vi "Finish.vi"   [LabVIEW 2015]
doc: "This VI is called just before exiting. It is expected to close I/O refnum, save collected data, etc."
uses:
  <vilib>/Rock Robotics/WPI/Utilities/WPI_GetSetVariantRefNum.vi
types:
  T1 = typedef "WPI_JoystickDevRef.ctl" = cluster{"Device":T2}
  T2 = typedef "WPI_JoystickDeviceEnum.ctl" = enum16{"USB 0", "USB 1", "USB 2", "USB 3", "USB 4", "USB 5"}
  T3 = typedef "WPI_CompressorDevRef.ctl" = cluster{"DevStatus":errorcluster, "Pneumatics Control Module":u8}
  T4 = typedef "WPI_EncoderDevRef.ctl" = cluster{"DevStatus":errorcluster, "EncoderIndex":T5, "CounterIndex":T6, "DistancePerCount":dbl, "Decoding Type":T7}
  T5 = typedef "FPGA_EncoderIdx.ctl" = enum8{"Enc 0", "Enc 1", "Enc 2", "Enc 3", "Enc 4", "Enc 5", "Enc 6", "Enc 7", "Invalid"}
  T6 = typedef "FPGA_CounterCtrSystemIndex.ctl" = enum8{"Ctr 0", "Ctr 1", "Ctr 2", "Ctr 3", "Ctr 4", "Ctr 5", "Ctr 6", "Ctr 7", "Invalid"}
  T7 = typedef "WPI_EncoderType.ctl" = enum16{"1x", "2x", "4x"}
  T8 = typedef "WPI_SolenoidDevRef.ctl" = cluster{"DevStatus":errorcluster, "Pneumatics Control Module":u8, "Forward Solenoid Channel":T9, "Reverse Solenoid Channel":T9}
  T9 = typedef "WPI_SolenoidChannel.ctl" = enum8{"Solenoid 0", "Solenoid 1", "Solenoid 2", "Solenoid 3", "Solenoid 4", "Solenoid 5", "Solenoid 6", "Solenoid 7", "Invalid"}
  T10 = typedef "WPI_ServoDeviceRef.ctl" = cluster{"DeviceStatus":errorcluster, "PWM Channel":T11, "DeadBand":T12}
  T11 = typedef "FPGA_DIOPWMChannel.ctl" = enum8{"PWM 0", "PWM 1", "PWM 2", "PWM 3", "PWM 4", "PWM 5", "PWM 6", "PWM 7", "PWM 8", "PWM 9", "PWM MXP 0", "PWM MXP 1", "PWM MXP 2", "PWM MXP 3", "PWM MXP 4", "PWM MXP 5", "PWM MXP 6", "PWM MXP 7", "PWM MXP 8", "PWM MXP 9", "Invalid"}
  T12 = typedef "WPI_PWMDeadband.ctl" = cluster{"Name":string, "maxPositivePwm":i32, "minPositivePwm":i32, "centerPwm":i32, "maxNegativePwm":i32, "minNegativePwm":i32, "angularRange":u16}
  T13 = typedef "WPI_SwitchDevRef.ctl" = cluster{"DevStatus":errorcluster, "DIO Channel":T14, "CntIndex":T6, "Normally Closed":bool}
  T14 = typedef "FPGA_DIOChannel.ctl" = enum8{"DIO 0", "DIO 1", "DIO 2", "DIO 3", "DIO 4", "DIO 5", "DIO 6", "DIO 7", "DIO 8", "DIO 9", "DIO MXP 0", "DIO MXP 1", "DIO MXP 2", "DIO MXP 3", "DIO MXP 4", "DIO MXP 5", "DIO MXP 6", "DIO MXP 7", "DIO MXP 8", "DIO MXP 9", "DIO MXP 10", "DIO MXP 11", "DIO MXP 12", "DIO MXP 13", "DIO MXP 14", "DIO MXP 15", "Invalid"}
  T15 = typedef "WPI_RobotDriveDevRef.ctl" = cluster{"DevStatus":errorcluster, "Motors[]":T16[], "Square Inputs":bool, "Max Output":dbl}
  T16 = typedef "WPI_MotorControlDeviceRef.ctl" = cluster{"DeviceStatus":errorcluster, "Type":T17, "PWM":cluster{"PWM Channel":T11, "DeadBand":T12}, "CAN":cluster{"Device Number":u8, "Control Mode":T18, "Semaphore":T19, "Max Vout":dbl, "TalonSRX Control Mode":T20}, "Invert":bool}
  T17 = typedef "WPI_MotorControlType.ctl" = enum16{"PWM", "CAN", "CANTalonSRX"}
  T18 = typedef "WPI_CANJaguar_ControlMode.ctl" = enum8{"Percent VBus", "Current", "Speed", "Position", "Voltage"}
  T19 = typedef "Semaphore RefNum" = refnum<k1>
  T20 = typedef "WPI_CANTalonSRX_APIControlMode.ctl" = enum8{"Percent VBus", "Speed", "Position", "Slave", "Unchanged / Invalid", "Voltage Compensation", "Current", "Motion Profile"}
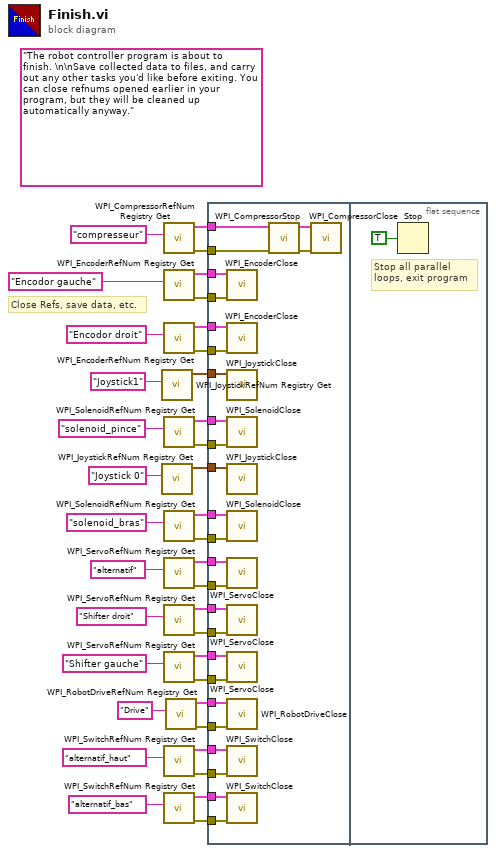
[diagram p0: block diagram]
diagram:
  (unwired) "The robot controller program is about to finish. \n\nSave collected data to files, and carry out any other tasks you'd like before exiting. You can close refnums opened earlier in your program, but they will be cleaned up automatically anyway."
  # "Close Refs, save data, etc."
  n1 = call <vilib>:"WPI_JoystickRefNum Registry Get.vi"("refnum name"="Joystick1") -> ("JoystickDevRef"=w22:T1)  [unwired: 1 in, 9 out]
  n2 = call <vilib>:"WPI_JoystickRefNum Registry Get.vi"("refnum name"="Joystick 0") -> ("JoystickDevRef"=w34:T1)  [unwired: 1 in, 9 out]
  n3 = call <vilib>:"WPI_CompressorRefNum Registry Get.vi"("refnum name"="compresseur") -> ("error out"=w16:errorcluster, "CompressorDevRef"=w17:T3)  [unwired: 9 in]
  n4 = call <vilib>:"WPI_EncoderRefNum Registry Get.vi"("refnum name"="Encodor gauche") -> ("error out"=w11:errorcluster, "EncoderDevRef"=w12:T4)  [unwired: 9 in]
  n5 = call <vilib>:"WPI_EncoderRefNum Registry Get.vi"("refnum name"="Encodor droit") -> ("error out"=w10:errorcluster, "EncoderDevRef"=w9:T4)  [unwired: 9 in]
  n6 = call <vilib>:"WPI_SolenoidRefNum Registry Get.vi"("refnum name"="solenoid_pince") -> ("error out"=w8:errorcluster, "SolenoidDevRef"=w18:T8)  [unwired: 9 in]
  n7 = call <vilib>:"WPI_SolenoidRefNum Registry Get.vi"("refnum name"="solenoid_bras") -> ("error out"=w7:errorcluster, "SolenoidDevRef"=w21:T8)  [unwired: 9 in]
  n8 = call <vilib>:"WPI_ServoRefNum Registry Get.vi"("refnum name"="alternatif") -> ("error out"=w1:errorcluster, "ServoDeviceRef"=w28:T10)  [unwired: 9 in]
  n9 = call <vilib>:"WPI_ServoRefNum Registry Get.vi"("refnum name"="Shifter droit") -> ("error out"=w6:errorcluster, "ServoDeviceRef"=w33:T10)  [unwired: 9 in]
  n10 = call <vilib>:"WPI_ServoRefNum Registry Get.vi"("refnum name"="Shifter gauche") -> ("error out"=w5:errorcluster, "ServoDeviceRef"=w32:T10)  [unwired: 9 in]
  n11 = call <vilib>:"WPI_SwitchRefNum Registry Get.vi"("refnum name"="alternatif_haut") -> ("error out"=w3:errorcluster, "SwitchDevRef"=w25:T13)  [unwired: 9 in]
  n12 = call <vilib>:"WPI_SwitchRefNum Registry Get.vi"("refnum name"="alternatif_bas") -> ("error out"=w4:errorcluster, "SwitchDevRef"=w24:T13)  [unwired: 9 in]
  n13 = call <vilib>:"WPI_RobotDriveRefNum Registry Get.vi"("refnum name"="Drive") -> ("error out"=w2:errorcluster, "RobotDriveDevRef"=w35:T15)  [unwired: 1 in, 8 out]
  n14 = flat-sequence {
    tunnel: w35 -> [w63]
    tunnel: w34 -> [w62]
    tunnel: w33 -> [w61]
    tunnel: w32 -> [w60]
    tunnel: w28 -> [w59]
    tunnel: w25 -> [w58]
    tunnel: w24 -> [w57]
    tunnel: w22 -> [w56]
    tunnel: w21 -> [w55]
    tunnel: w18 -> [w54]
    tunnel: w17 -> [w51]
    tunnel: w16 -> [w50]
    tunnel: w12 -> [w49]
    tunnel: w11 -> [w48]
    tunnel: w10 -> [w47]
    tunnel: w9 -> [w46]
    tunnel: w8 -> [w45]
    tunnel: w7 -> [w44]
    tunnel: w6 -> [w43]
    tunnel: w5 -> [w42]
    tunnel: w4 -> [w41]
    tunnel: w3 -> [w40]
    tunnel: w2 -> [w39]
    tunnel: w1 -> [w38]
    frame #0 {
      n15 = call <vilib>:"WPI_EncoderClose.vi"("error in (no error)"=w48, "EncoderDevRef"=w49) -> ()  [unwired: 9 in, 1 out]
      n16 = call <vilib>:"WPI_EncoderClose.vi"("error in (no error)"=w47, "EncoderDevRef"=w46) -> ()  [unwired: 9 in, 1 out]
      n17 = call <vilib>:"WPI_JoystickClose.vi"("JoystickDevRef"=w56) -> ()  [unwired: 11 out]
      n18 = call <vilib>:"WPI_SolenoidClose.vi"("error in (no error)"=w45, "SolenoidDevRef"=w54) -> ()  [unwired: 9 in, 1 out]
      n19 = call <vilib>:"WPI_JoystickClose.vi"("JoystickDevRef"=w62) -> ()  [unwired: 11 out]
      n20 = call <vilib>:"WPI_SolenoidClose.vi"("error in (no error)"=w44, "SolenoidDevRef"=w55) -> ()  [unwired: 9 in, 1 out]
      n21 = call <vilib>:"WPI_ServoClose.vi"("error in (no error)"=w38, "ServoDeviceRef"=w59) -> ()  [unwired: 9 in, 1 out]
      n22 = call <vilib>:"WPI_ServoClose.vi"("error in (no error)"=w43, "ServoDeviceRef"=w61) -> ()  [unwired: 9 in, 1 out]
      n23 = call <vilib>:"WPI_ServoClose.vi"("error in (no error)"=w42, "ServoDeviceRef"=w60) -> ()  [unwired: 9 in, 1 out]
      n24 = call <vilib>:"WPI_RobotDriveClose.vi"("error in (no error)"=w39, "RobotDriveDevRef"=w63) -> ()  [unwired: 10 out]
      n25 = call <vilib>:"WPI_SwitchClose.vi"("error in (no error)"=w40, "SwitchDevRef"=w58) -> ()  [unwired: 9 in, 1 out]
      n26 = call <vilib>:"WPI_SwitchClose.vi"("error in (no error)"=w41, "SwitchDevRef"=w57) -> ()  [unwired: 9 in, 1 out]
      n27 = call <vilib>:"WPI_CompressorStop.vi"("error in (no error)"=w50, "CompressorDevRef"=w51) -> ("error out"=w53:errorcluster, "CompressorDevRef"=w52:T3)  [unwired: 8 in]
      n28 = call <vilib>:"WPI_CompressorClose.vi"("error in (no error)"=w53, "CompressorDevRef"=w52) -> ()  [unwired: 9 in, 1 out]
    }
    frame #1 {
      # "Stop all parallel\nloops, exit program"
      n29 = Stop(stop? (T)=TRUE ("Quit")) -> ()
    }
  }
